vi "Change VI Description.vi"(6 "VI Path":path, 7 "Assert Scripting Configuration":T1={"Assert Name"="", "Comment"="", "Numeric Operation"="", "Type"=enum."Double Float", "String Operation"="", "DBL Comparison Value 1"=0.0, "DBL Comparison Value 2"=0.0, "I32 Comparison Value 1"=0, "I32 Comparison Value 2"=0, "Creator"="", "Creation Timestamp"=timestamp(0 s since 1904-01-01), "String Comparison Value"="", "Description"="", "Default Failure Action"=enum."None", "Boolean Comparison Value"=FALSE}, 8 "error in (no error)":errorcluster, 10 "Evaluation String":string) -> (0 "error out":errorcluster)   [LabVIEW 2016]
uses:
  Assert Scripting Configuration.ctl
  <vilib>/Utility/Data Type/Type Definitions/Data Type.ctl
  <vilib>/Utility/Data Type/NI_Data Type.lvlib
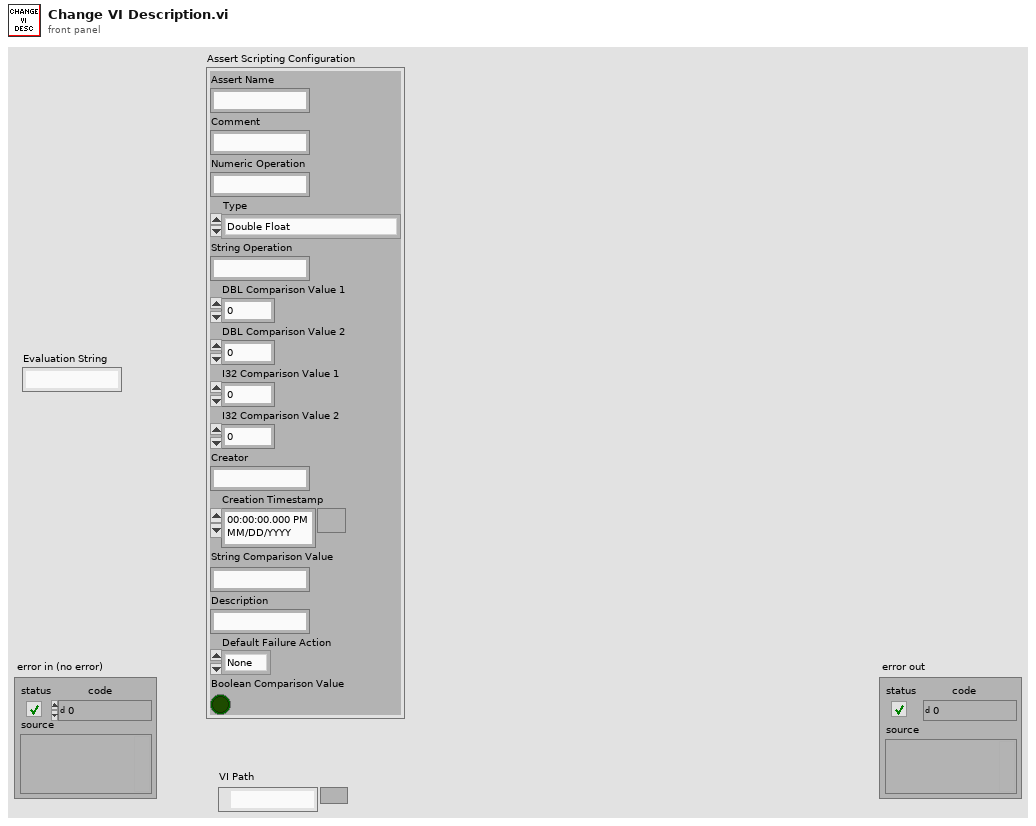
[diagram p1: front panel]
types:
  T1 = typedef "Assert Scripting Configuration.ctl" = cluster{"Assert Name":string, "Comment":string, "Numeric Operation":string, "Type":T2, "String Operation":string, "DBL Comparison Value 1":dbl, "DBL Comparison Value 2":dbl, "I32 Comparison Value 1":i32, "I32 Comparison Value 2":i32, "Creator":string, "Creation Timestamp":timestamp, "String Comparison Value":string, "Description":string, "Default Failure Action":enum16{"None", "Log To File", "Pause Execution", "Abort Execution"}, "Boolean Comparison Value":bool}
  T2 = typedef "NI_Data Type.lvlib/Data Type.ctl" = enum8{"Invalid Type", "Void", "I8", "I16", "I32", "I64", "U8", "U16", "U32", "U64", "Single Float", "Double Float", "Extended Float", "Single Complex", "Double Complex", "Extended Complex", "Enum U8", "Enum U16", "Enum U32", "Enum U64", "Single Float With Unit", "Double Float With Unit", "Extended Float With Unit", "Single Complex with Unit", "Double Complex with Unit", "Extended Complex with Unit", "Boolean", "String", "Path", "Picture", "Tag", "Array", "Cluster", "Variant", "LV Variant", "Waveform", "Timestamp", "Digital Waveform", "Digital Data", "ExpressData", "Refnum", "External Data", "VI", "Poly VI", "LabVIEW Class Instance", "Fixed Point"}
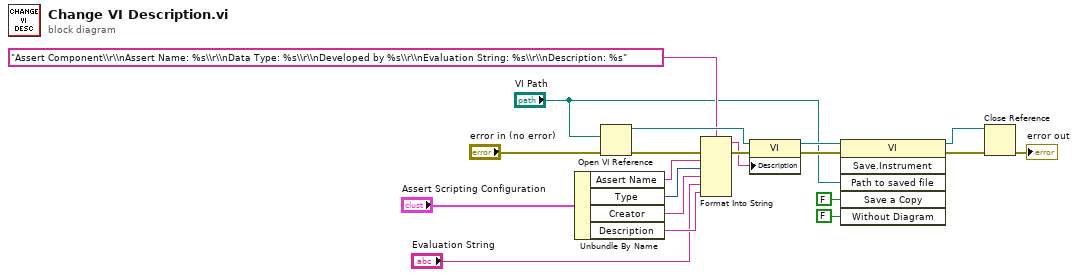
[diagram p0: block diagram]
diagram:
  n1 = Unbundle By Name("Assert Scripting Configuration") -> ("Assert Name"=w13:string, "Type"=w12:T2, "Creator"=w11:string, "Description"=w10:string)
  n2 = Open VI Reference(vi path="VI Path", error in (no error)="error in (no error)") -> (vi reference=w19:refnum<vi>, error out=w18:errorcluster)  [unwired: 4 in]
  n3 = Format Into String(format string="Assert Component\\r\\nAssert Name: %s\\r\\nData Type: %s\\r\\nDeveloped by %s\\r\\nEvaluation String: %s\\r\\nDescription: %s", error in=w18, w13, w12, w11, "Evaluation String", w10) -> (resulting string=w8:string, error out=w14:errorcluster)  [unwired: 1 in]
  n4 = property class="VI"(reference=w19, error in=w14, "Description"=w8) -> (reference out=w6:refnum<vi>, error out=w17:errorcluster)
  n5 = invoke class="VI" method="Save.Instrument"(reference=w6, error in=w17, "Path to saved file"="VI Path", "Save a Copy"=FALSE, "Without Diagram"=FALSE) -> (reference out=w5:refnum<vi>, error out=w7:errorcluster)  [unwired: 1 in, 4 out]
  n6 = Close Reference(reference=w5, error in (no error)=w7) -> (error out=→"error out":errorcluster)
